vi "Delete Attributes.vi"(7 "ID":string, 8 "error in (no error)":errorcluster, 9 "Attributes":variant[](array[variant]), 10 "Attribute Names":string[](array[string]), 11 "Test Executive in":refnum<class "Test Executive.lvclass">) -> (0 "error out":errorcluster, 1 "Found":bool, 3 "Test Executive out":refnum<class "Test Executive.lvclass">)   [LabVIEW 2017, in "Test Executive.lvlib" / "Test Executive.lvclass"]
uses:
  <vilib>/gpm_packages/@cs/test-executive/Source/Test Executive/TestExecutive/Test Executive.lvclass
  <vilib>/gpm_packages/@cs/test-executive/Source/Test Executive/TestExecutive/Test Executive.lvclass/Test Executive.ctl
  779bede0-b176-4fbf-b39a-2c4718ecdec0.vi
  <vilib>/gpm_packages/@cs/linked-list/Source/Linked List/ILinkedList/ILinked List.lvclass
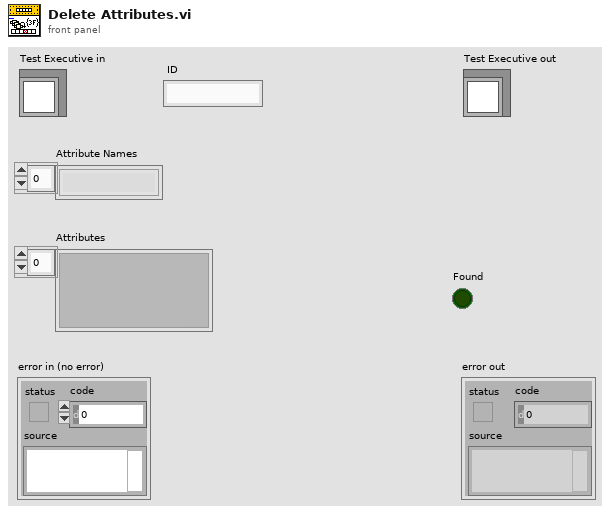
[diagram p1: front panel]
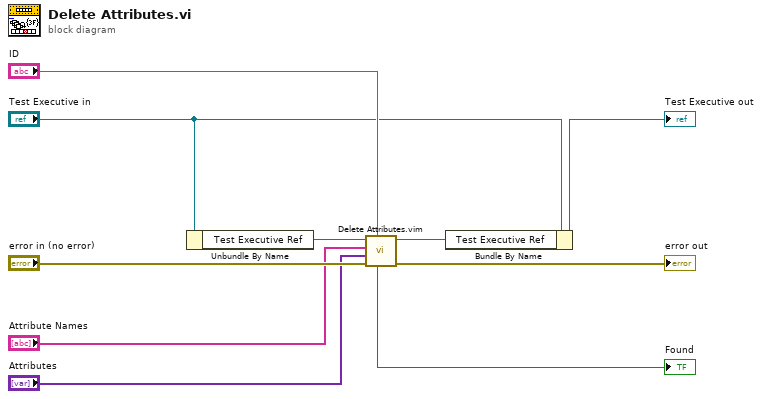
[diagram p0: block diagram]
diagram:
  n1 = Unbundle By Name("Test Executive in") -> ("Test Executive Ref"=w6:refnum<data-value>)
  n2 = call "Delete Attributes.vim"("Linked List ID"="ID", "error in (no error)"="error in (no error)", "Types"="Attributes", "Attribute Names"="Attribute Names", "Linked List Ref"=w6) -> ("error out"=→"error out":errorcluster, "Linked List Ref out"=w5:refnum<data-value>, "Found?"=→"Found":bool)  [unwired: 4 in]
  n3 = Bundle By Name(cluster="Test Executive in", "Test Executive Ref"=w5) -> (→"Test Executive out":refnum<class "Test Executive.lvclass">)
